vi "Stop Measurement.vi"(8 "error in (no error)":errorcluster, 10 "Measurement name":string, 11 "Mag Lab Measure Controller in":refnum<class "Mag Lab Measure Controller.lvclass">) -> (0 "error out":errorcluster, 3 "Mag Lab Measure Controller out":refnum<class "Mag Lab Measure Controller.lvclass">)   [LabVIEW 2015, in "Mag Lab Measure Controller.lvclass"]
uses:
  Mag Lab Measure Controller.lvclass
  Mag Lab Root/Mag Lab Root.lvclass/Mag Lab Root.ctl
  Mag Lab Measure Controller.lvclass/Mag Lab Measure Controller.ctl
  Mag Lab Root Messages/Halt Msg/Halt Msg.lvclass/Halt Msg.ctl
  <vilib>/ActorFramework/Message Enqueuer/Message Enqueuer.lvclass/Message Enqueuer.ctl
  <vilib>/ActorFramework/Message Enqueuer/Enqueue.vi
  <vilib>/ActorFramework/Message Priority Queue/Priority Enqueue.vi
  Mag Lab Root Messages/Halt Msg/Halt Msg.lvclass
  Mag Lab Root/Mag Lab Root.lvclass
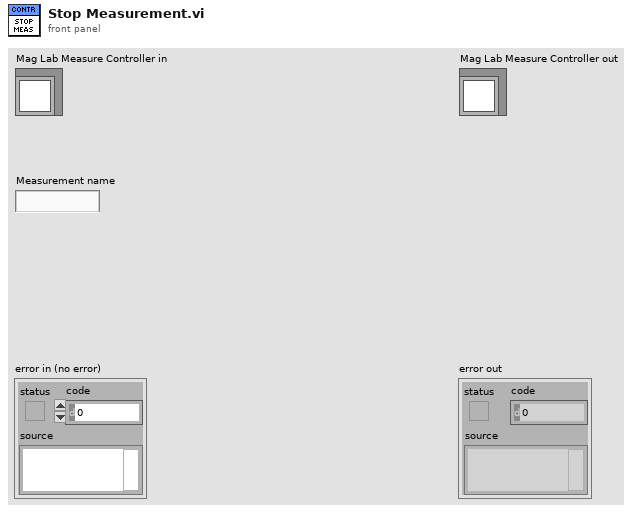
[diagram p1: front panel]
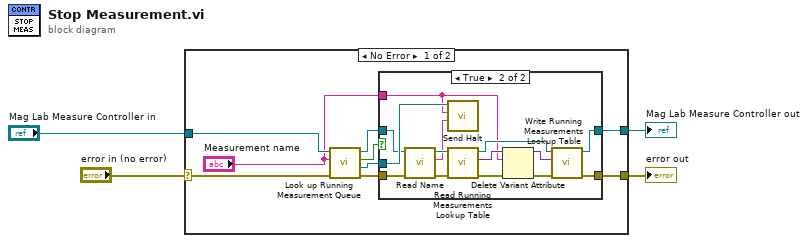
[diagram p0: block diagram]
diagram:
  n1 = case shown="No Error" "error in (no error)" {
    selector: "error in (no error)" -> [w5 w31]
    tunnel: [w7 w31] -> w3
    tunnel: [w6 w30] -> w1
    tunnel: "Mag Lab Measure Controller in" -> [w13 w30]
    frame No Error {
      n2 = call "Look up Running Measurement Queue .vi"("error in (no error)"=w5, "Measurement Name.Harware()"="Measurement name", "Mag Lab Measure Controller in"=w13) -> ("error out"=w8:errorcluster, "Measurement Queue"=w11:refnum<class "Message Enqueuer.lvclass">, "Found?"=w12:bool, "Mag Lab Measure Controller out"=w10:refnum<class "Mag Lab Measure Controller.lvclass">)  [unwired: 4 in]
      n3 = case shown="True" w12 {
        tunnel: w11 -> [_ w22]
        tunnel: w10 -> [w15 w20]
        tunnel: "Measurement name" -> [_ w21]
        tunnel: w8 -> [w14 w18]
        tunnel: [w14 w24] -> w7
        tunnel: [w15 w23] -> w6
        frame False {
        }
        frame True {
          n4 = call "Read Name.vi"("error in (no error)"=w18, "Mag Lab Root in"=w20) -> ("error out"=w17:errorcluster, "Name"=w16:string, "Mag Lab Root out"=w19:refnum<class "Mag Lab Measure Controller.lvclass">)  [unwired: 7 in]
          n5 = call "Send Halt.vi"("Requestor"=w16, "Requestee"=w21, "Message Enqueuer"=w22) -> ()  [unwired: 7 in, 2 out]
          n6 = call "Read Running Measurements Lookup Table.vi"("error in (no error)"=w17, "Mag Lab Measure Controller in"=w19) -> ("error out"=w25:errorcluster, "Running Measurements Queue Lookup Table"=w29:variant, "Mag Lab Measure Controller out"=w28:refnum<class "Mag Lab Measure Controller.lvclass">)  [unwired: 7 in]
          n7 = Delete Variant Attribute(4:w25, 6:w21, 7:w29) -> (0:w26:errorcluster, 3:w27:variant)  [unwired: 1 out]
          n8 = call "Write Running Measurements Lookup Table.vi"("error in (no error)"=w26, "Running Measurements Queue Lookup Table"=w27, "Mag Lab Measure Controller in"=w28) -> ("error out"=w24:errorcluster, "Mag Lab Measure Controller out"=w23:refnum<class "Mag Lab Measure Controller.lvclass">)  [unwired: 7 in]
        }
      }
    }
    frame Error {
    }
  }
  "error out" <- w3
  "Mag Lab Measure Controller out" <- w1
